vi "Write_UI2R_to_File.vi"(8 "error in (no error)":errorcluster, 9 "ControlValueUpdates[]":T1[](array[typedef]), 10 "UI2R Save Filepath":path, 11 "UI_Interaction_Manager in":refnum<class "UI_Interaction_Manager.lvclass">) -> (0 "error out":errorcluster, 3 "UI_Interaction_Manager out":refnum<class "UI_Interaction_Manager.lvclass">)   [LabVIEW 2011, in "UI_Interaction_Manager.lvclass"]
uses:
  UI_Interaction_Manager.lvclass
  TypeDefs/ControlValueUpdate.ctl
  TypeDefs/UI_Interaction_Record.ctl
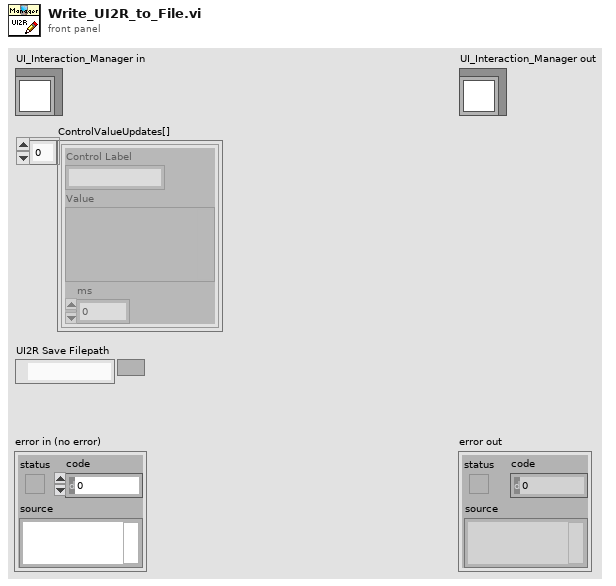
[diagram p1: front panel]
types:
  T1 = typedef "UI_Interaction_Manager.lvclass/ControlValueUpdate.ctl" = cluster{"Control Label":string, "Value":variant, "ms":u32}
  T2 = enum16{"open", "replace", "create", "open or create", "replace or create", "replace or create with confirmation"}
  T3 = typedef "UI_Interaction_Manager.lvclass/UI_Interaction_Record.ctl" = cluster{"UI Filepath":path, "Recorded Events":T1[]}
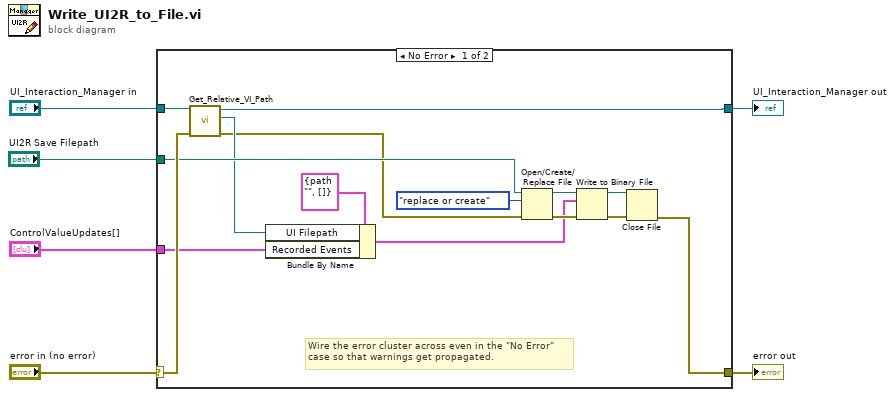
[diagram p0: block diagram]
diagram:
  n1 = case shown="No Error" "error in (no error)" {
    selector: "error in (no error)" -> [w13 w23]
    tunnel: [w11 w23] -> w5
    tunnel: [w14 w22] -> w3
    tunnel: "UI_Interaction_Manager in" -> [w15 w22]
    tunnel: "ControlValueUpdates[]" -> [w12 _]
    tunnel: "UI2R Save Filepath" -> [w10 _]
    frame No Error {
      # "Wire the error cluster across even in the \"No Error\"\ncase so that warnings get propagated."
      n2 = call "Get_Relative_VI_Path.vi"("error in (no error)"=w13, "UI_Interaction_Manager in"=w15) -> ("error out"=w7:errorcluster, "Relative VI Path"=w9:path, "UI_Interaction_Manager out"=w14:refnum<class "UI_Interaction_Manager.lvclass">)  [unwired: 7 in]
      n3 = Bundle By Name(cluster=T3 {"UI Filepath"=path "", "Recorded Events"=[]} ("Cluster"), "UI Filepath"=w9, "Recorded Events"=w12) -> (w8:T3)
      n4 = Open/Create/Replace File(file path (use dialog)=w10, error in=w7, operation (0:open)=T2."replace or create") -> (refnum out=w17:refnum<file>, error out=w18:errorcluster)  [unwired: 3 in, 1 out]
      n5 = Write to Binary File(file (use dialog)=w17, data=w8, error in=w18) -> (refnum out=w20:refnum<file>, error out=w19:errorcluster)  [unwired: 3 in, 1 out]
      n6 = Close File(refnum=w20, error in=w19) -> (error out=w11:errorcluster)  [unwired: 1 out]
    }
    frame Error {
    }
  }
  "error out" <- w5
  "UI_Interaction_Manager out" <- w3
